vi "Wait for Spark Global.vi"(4 "Timeout (ms)":i32) -> (1 "Spark!":bool)   [LabVIEW 2012]
uses:
  C/LabVIEW for MTA/DaveP/LabVIEW Development/LabVIEW 2012 versions/Dave's Test VIs/DWP Scope VIs/201 MHz Global Cavity Variables.vi
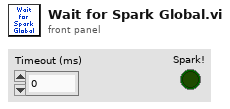
[diagram p1: front panel]
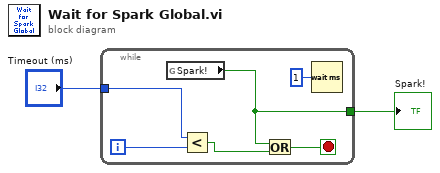
[diagram p0: block diagram]
diagram:
  n1 = while {
    tunnel: "Timeout (ms)" -> [w6]
    tunnel: [w3] -> w1
    i -> [w4]
    stop <- w7 stop-if-true
    n2 = global read "201 MHz Global Cavity Variables.vi" "Spark!"() -> (w3:bool)
    n3 = Less?(x=w6, y=w4) -> (x < y?=w5:bool)
    n4 = Or(x=w3, y=w5) -> (x .or. y?=w7:bool)
    n5 = Wait (ms)(milliseconds to wait=u32 1) -> ()  [unwired: 1 out]
  }
  "Spark!" <- w1
